vi "ps_configure.vi"(8 "error in (no error)":errorcluster, 10 "SET PS":T1, 11 "Instrument in":refnum<class "Instrument.lvclass">) -> (0 "error out":errorcluster, 3 "Instrument out":refnum<class "Instrument.lvclass">)   [LabVIEW 2019, in "Instrument.lvclass"]
uses:
  Instrument.lvclass
  Instrument.lvclass/Instrument.ctl
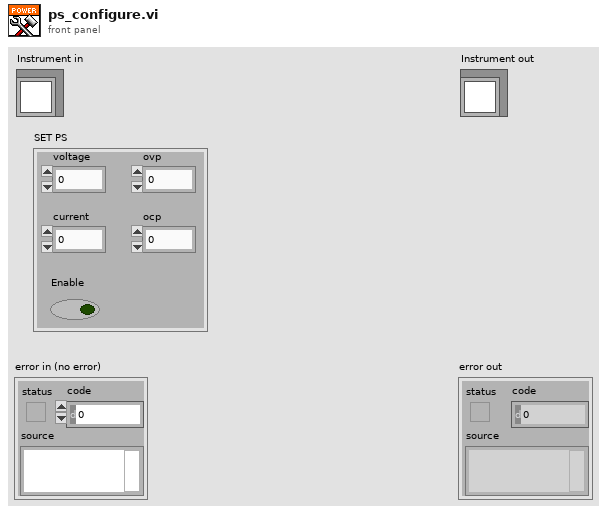
[diagram p1: front panel]
types:
  T1 = cluster{"voltage":sgl, "current":sgl, "ovp":sgl, "ocp":sgl, "Enable":bool}
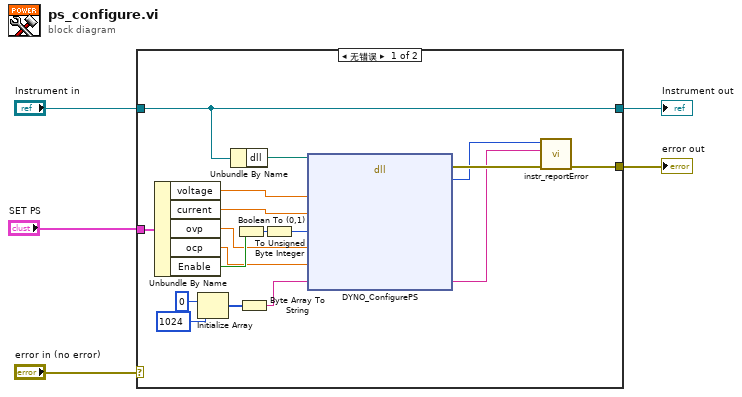
[diagram p0: block diagram]
diagram:
  n1 = case shown="无错误" "error in (no error)" {
    selector: "error in (no error)" -> [_ w25]
    tunnel: [w14 w25] -> w4
    tunnel: [w23 w24] -> w2
    tunnel: "Instrument in" -> [w23 w24]
    tunnel: "SET PS" -> [w11 _]
    frame No Error {
      n2 = Unbundle By Name(w11) -> ("voltage"=w6:sgl, "current"=w7:sgl, "ovp"=w8:sgl, "ocp"=w9:sgl, "Enable"=w10:bool)
      n3 = Initialize Array(u8 0 ("element"), 1024 ("dimension size")) -> (w18:u8[])
      n4 = Unbundle By Name(w23) -> ("dll"=w22:path)
      n5 = Boolean To (0,1)(Boolean=w10) -> (0, 1=w21:i16)
      n6 = Byte Array To String(unsigned byte array=w18) -> (string=w17:string)
      n7 = To Unsigned Byte Integer(number=w21) -> (unsigned 8bit integer=w16:u8)
      n8 = dll-call lib="C:/Dev/22KW-Dyno/software/data/DynoAPI.dll" fn="DYNO_ConfigurePS"(path in=w22, "voltage"=w6, "current"=w7, "enable"=w16, "ovp"=w8, "ocp"=w9, "errorMsg"=w17) -> (error out=w15:errorcluster, "return type"=w13:i32, "errorMsg"=w12:string)  [unwired: 7 in, 1 out]
      n9 = call "instr_reportError.vi"("error in (no error)"=w15, "errorMsg"=w12, "return type"=w13) -> ("error out"=w14:errorcluster)  [unwired: 8 in]
    }
    frame Error {
    }
  }
  "error out" <- w4
  "Instrument out" <- w2
